vi "FPGAFilter_subCU.vi"(8 "states":cluster{"addr start":u16, "first run?":bool}, 9 "global reset":bool, 10 "filter length":i32=1000, 11 "index":u16) -> (0 "states":cluster{"addr start":u16, "first run?":bool}, 1 "control info":T1)   [LabVIEW 2023]
panel:
  in  "control info 2":T1
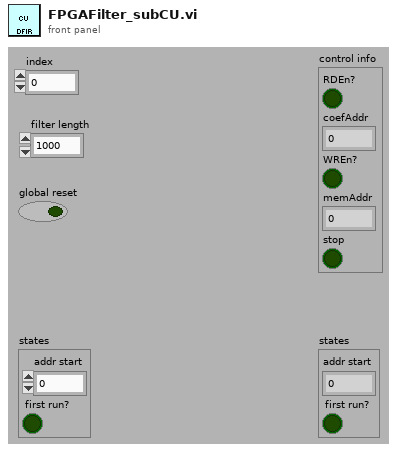
[diagram p1: front panel]
types:
  T1 = cluster{"RDEn?":bool, "coefAddr":u16, "WREn?":bool, "memAddr":u16, "stop":bool}
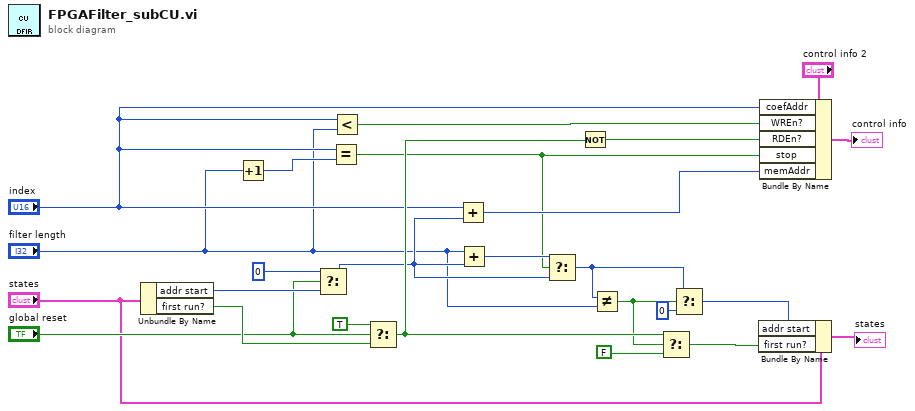
[diagram p0: block diagram]
diagram:
  n1 = Unbundle By Name("states") -> ("addr start"=w24:u16, "first run?"=w25:bool)
  n2 = Increment(x="filter length") -> (x+1=w2:i32)
  n3 = Select(t=u16 0, s="global reset", f=w24) -> (s? t:f=w17:u16)
  n4 = Equal?(x="index", y=w2) -> (x = y?=w3:bool)
  n5 = Less?(x="index", y="filter length") -> (x < y?=w6:bool)
  n6 = Select(t=TRUE, s="global reset", f=w25) -> (s? t:f=w22:bool)
  n7 = Add(x="index", y=w17) -> (x+y=w4:u16)
  n8 = Add(x="filter length", y=w17) -> (x+y=w15:i32)
  n9 = Select(t=w15, s=w3, f=w17) -> (s? t:f=w16:i32)
  n10 = Not(x=w22) -> (.not. x?=w7:bool)
  n11 = Not Equal?(x=w16, y="filter length") -> (x != y?=w19:bool)
  n12 = Select(t=w22, s=w19, f=FALSE ("t")) -> (s? t:f=w23:bool)
  n13 = Select(t=w16, s=w19, f=u16 0) -> (s? t:f=w9:i32)
  n14 = Bundle By Name(cluster="states", "addr start"=w9, "first run?"=w23) -> (→"states":cluster{"addr start":u16, "first run?":bool})
  n15 = Bundle By Name(cluster="control info 2", "coefAddr"="index", "WREn?"=w6, "RDEn?"=w7, "stop"=w3, "memAddr"=w4) -> (→"control info":T1)
